vi "pH_FGV.vi"(7 "Command":enum16{"SET", "GET"}(ring), 8 "error in (no error)":errorcluster, 10 "Elapsed_Time(s)":dbl, 11 "pH_Value_IN":dbl) -> (0 "error out":errorcluster, 2 "Elapsed_Time(s)_OUT":dbl, 3 "pH_Value_OUT":dbl)   [LabVIEW 2017]
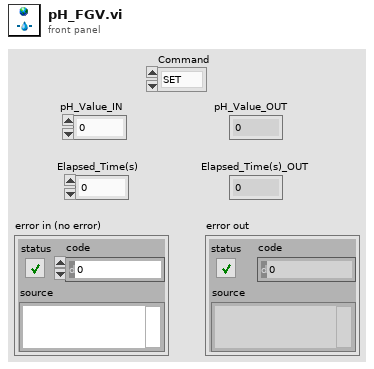
[diagram p1: front panel]
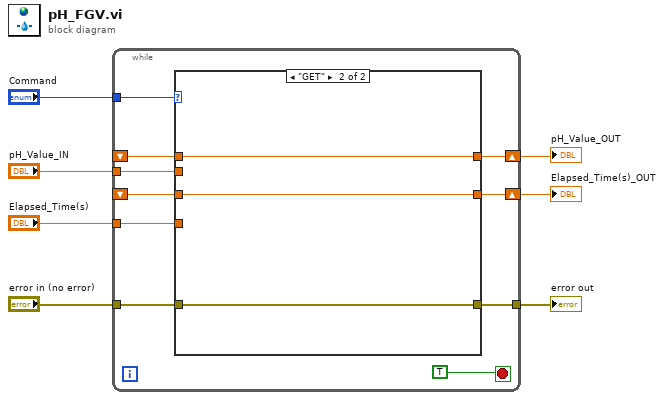
[diagram p0: block diagram]
diagram:
  n1 = while {
    tunnel: "Command" -> [w17]
    shift-right: [w16] -> w6
    shift-left: _ -> [w12]
    shift-right: [w14] -> w5
    shift-left: _ -> [w11]
    tunnel: "pH_Value_IN" -> [w15]
    tunnel: "Elapsed_Time(s)" -> [w13]
    tunnel: [w9] -> w2
    tunnel: "error in (no error)" -> [w8]
    stop <- TRUE stop-if-true
    n2 = case shown="\"GET\"" w17 {
      tunnel: [w20 w23] -> w16
      tunnel: w15 -> [w20 _]
      tunnel: [w19 w22] -> w14
      tunnel: w13 -> [w19 _]
      tunnel: w12 -> [_ w23]
      tunnel: w11 -> [_ w22]
      tunnel: [w18 w21] -> w9
      tunnel: w8 -> [w18 w21]
      frame "SET", Default {
      }
      frame "GET" {
      }
    }
  }
  "pH_Value_OUT" <- w6
  "Elapsed_Time(s)_OUT" <- w5
  "error out" <- w2
